vi "Exercise 1.4 PWM.vi"(8 "error in (no error)":errorcluster) -> (0 "error out":errorcluster)   [LabVIEW 2014]
uses:
  <vilib>/Q-Wave Systems/QwaveSys RPi Training Package (Demo)/Addons/QwaveSys RPi Training Library.lvlib
panel:
  out "PWM RAW Output":i32(knob)=862 scale=0.0..300.0
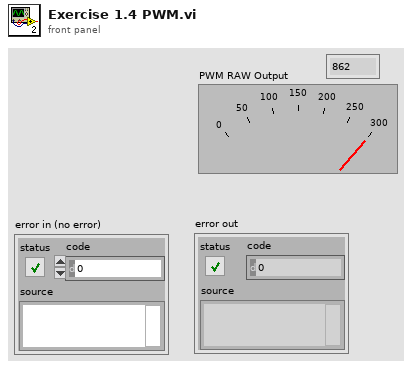
[diagram p1: front panel]
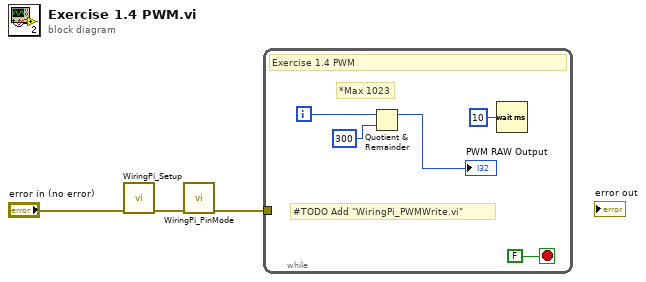
[diagram p0: block diagram]
diagram:
  n1 = call <vilib>:"WiringPi_Setup.vi"("error in (no error)"="error in (no error)") -> ("error out"=w2:errorcluster)  [unwired: 10 in]
  n2 = call <vilib>:"WiringPi_PinMode.vi"("error in (no error)"=w2) -> ("error out"=w1:errorcluster)  [unwired: 10 in]
  n3 = while {
    tunnel: w1 -> [_]
    i -> [w5]
    stop <- FALSE stop-if-true
    # "#TODO Add \"WiringPi_PWMWrite.vi\""
    # "*Max 1023"
    # "Exercise 1.4 PWM"
    n4 = Quotient & Remainder(x=w5, y=300) -> (x-y*floor(x/y)=→"PWM RAW Output":i32)  [unwired: 1 out]
    n5 = Wait (ms)(milliseconds to wait=u32 10) -> ()  [unwired: 1 out]
  }
